vi "Find Row Index from Property Name.vi"(8 "错误输入":cluster{"状态":bool, "代码":i32, "源":string}, 10 "属性名":string, 11 "电子表格字符串数组":string[][](array[string])) -> (0 "错误输出":cluster{"状态":bool, "代码":i32, "源":string}, 2 "行索引":i32, 3 "电子表格字符串数组输出":string[][](array[string]))   [LabVIEW 2012]
doc: "对于给定的搜索字符串，搜索第0列构成的字符串数组（通常是程序打开的一个文本文件），返回行索引。"
uses:
  <vilib>/Utility/error.llb/Error Cluster From Error Code.vi
  <vilib>/ErrorRing/Error Ring.xnode
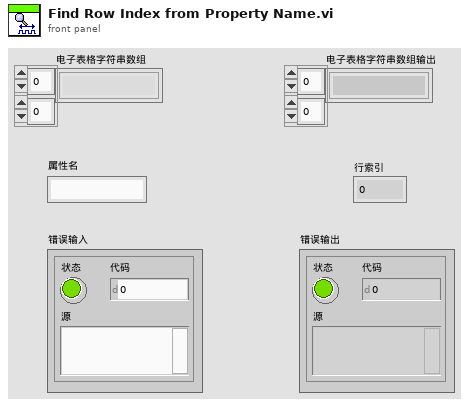
[diagram p1: front panel]
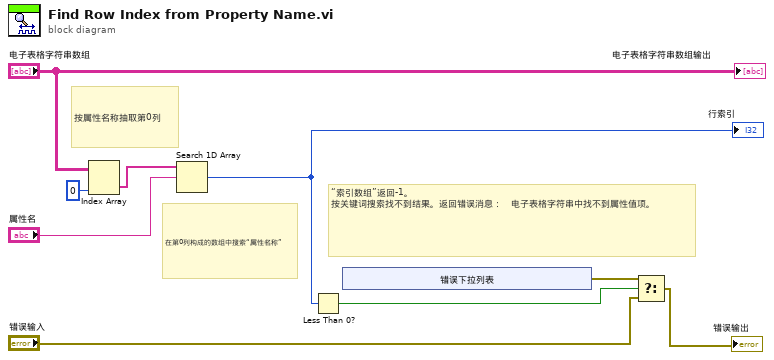
[diagram p0: block diagram]
diagram:
  # "“索引数组”返回-1。\n按关键词搜索找不到结果。返回错误消息：   电子表格字符串中找不到属性值项。"
  # "在第0列构成的数组中搜索“属性名称”"
  # "按属性名称抽取第0列"
  n1 = Index Array ("索引数组")(array="电子表格字符串数组", index (col)=0 ("禁用索引（列）")) -> (element=w8:string[])  [unwired: 1 in]
  n2 = Search 1D Array ("搜索一维数组")(1D array=w8, element="属性名") -> (index of element=w5:i32)  [unwired: 1 in]
  "行索引" <- w5
  n3 = Less Than 0? ("小于0？")(x=w5) -> (x < 0?=w4:bool)
  n4 = xnode "错误下拉列表"() -> ("错误输出"=w2:errorcluster)
  n5 = Select ("选择")(t=w2, s=w4, f="错误输入") -> (s? t:f=→"错误输出":cluster{"状态":bool, "代码":i32, "源":string})
  "电子表格字符串数组输出" <- "电子表格字符串数组"
